vi "RP Lockin Fast Continuous Sweeper.vi"(6 "Samples per read":i32=1024, 7 "Desimate result":i32, 8 "Error In":errorcluster, 10 "Frequencies":dbl[](array[numeric]), 11 "connection ID":refnum<k5>) -> (0 "Error Out":errorcluster, 1 "Y":dbl[](array[numeric]), 2 "X":dbl[](array[numeric]), 3 "connection ID out":refnum<k5>, 4 "F":dbl[](array[numeric]))   [LabVIEW 2015]
panel:
  out "Input Fifo cnt 2":i32
  out "32bit integer":i32
  out "Output Fifo cnt":i32
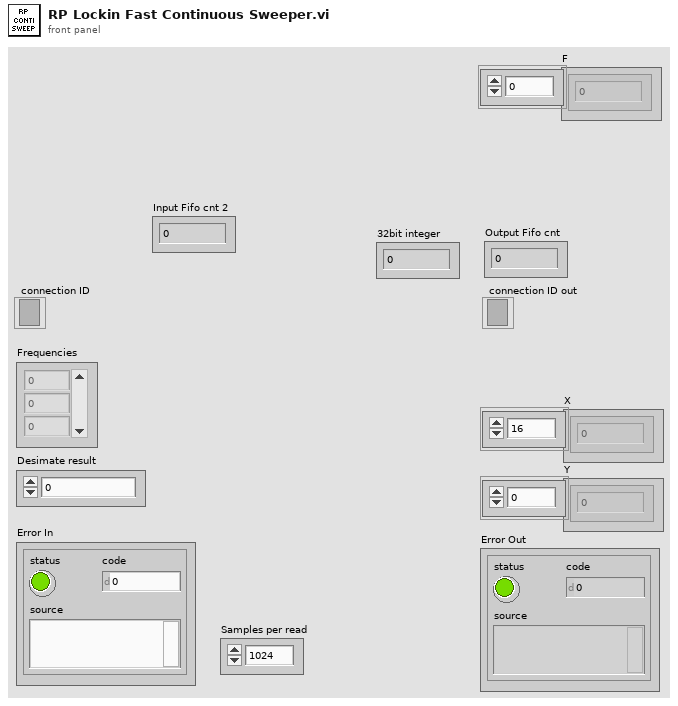
[diagram p1: front panel]
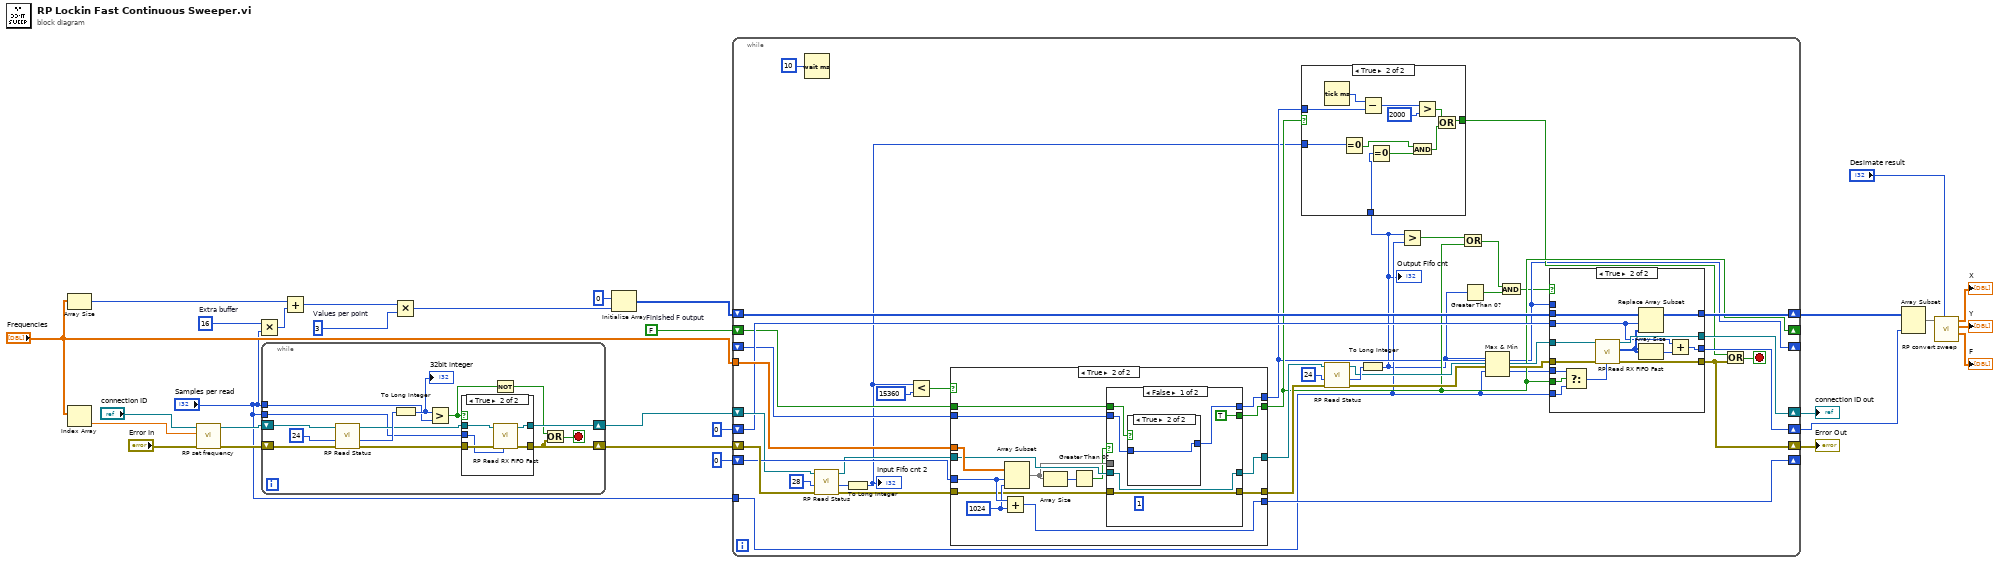
[diagram p0: block diagram]
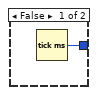
[diagram p5: hidden frame]
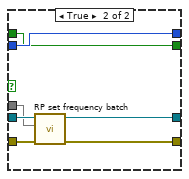
[diagram p6: hidden frame]
diagram:
  w13 = 3  # Values per point
  w16 = 16  # Extra buffer
  w19 = FALSE  # Finished F output
  n1 = Array Size(array="Frequencies") -> (size(s)=w17:i32)
  n2 = Index Array(array="Frequencies") -> (element=w29:dbl)  [unwired: 1 in]
  n3 = call "RP set frequency.vi"("Error In"="Error In", "Frequency"=w29, "connection ID"="connection ID") -> ("Error Out"=w23:errorcluster, "connection ID out"=w25:refnum<k5>)  [unwired: 6 in, 1 out]
  n4 = Multiply(x=w16, y="Samples per read") -> (x*y=w15:i32)
  n5 = while {
    tunnel: "Samples per read" -> [w40]
    shift-right: [w30] -> w22
    shift-left: w23 -> [w37]
    shift-right: [w35] -> w24
    shift-left: w25 -> [w36]
    tunnel: "Samples per read" -> [w34]
    stop <- w33 stop-if-true
    n6 = call "RP Read Status.vi"("Error In"=w37, "Status offset"=u64 24, "connection ID"=w36) -> ("Error Out"=w32:errorcluster, "Status response"=w41:u32, "connection ID out"=w39:refnum<k5>)  [unwired: 6 in]
    n7 = To Long Integer(number=w41) -> (32bit integer=w42:i32)
    "32bit integer" <- w42
    n8 = Greater?(x=w42, y=w40) -> (0:w38:bool)
    n9 = case shown="True" w38 {
      tunnel: w39 -> [w45 w50]
      tunnel: w32 -> [w44 w49]
      tunnel: [w44 w48] -> w30
      tunnel: [w45 w47] -> w35
      tunnel: w34 -> [_ w46]
      frame False {
      }
      frame True {
        n10 = call "RP Read RX FIFO Fast.vi"("Samples per read"=w46, "Error In"=w49, "connection ID"=w50) -> ("Error Out"=w48:errorcluster, "connection ID out"=w47:refnum<k5>)  [unwired: 6 in, 1 out]
      }
    }
    n11 = Not(x=w38) -> (.not. x?=w31:bool)
    n12 = Or(x=w31, y=w30) -> (x .or. y?=w33:bool)
  }
  n13 = Add(x=w17, y=w15) -> (x+y=w14:i32)
  n14 = Multiply(x=w14, y=w13) -> (x*y=w11:i32)
  n15 = Initialize Array(0, w11) -> (w10:i32[])
  n16 = while {
    tunnel: "Frequencies" -> [w88]
    tunnel: "Samples per read" -> [w53]
    shift-right: [w62] -> w20
    shift-left: w22 -> [w87]
    shift-right: [w86] -> w26
    shift-left: w24 -> [w70]
    shift-right: [w83] -> _
    shift-left: 0 -> [w84]
    shift-right: [w59] -> _
    shift-left: w19 -> [w60]
    shift-right: [w65] -> w8
    shift-left: w10 -> [w68]
    shift-right: [w66] -> w5
    shift-left: 0 -> [w67]
    shift-right: [w57] -> _
    shift-left: _ -> [w61]
    stop <- w85 stop-if-true
    n17 = Wait (ms)(milliseconds to wait=u32 10) -> ()  [unwired: 1 out]
    n18 = call "RP Read Status.vi"("Error In"=w87, "Status offset"=u64 28, "connection ID"=w70) -> ("Error Out"=w74:errorcluster, "Status response"=w78:u32, "connection ID out"=w73:refnum<k5>)  [unwired: 6 in]
    n19 = To Long Integer(number=w78) -> (32bit integer=w51:i32)
    "Input Fifo cnt 2" <- w51
    n20 = Less?(x=w51, y=15360) -> (x < y?=w75:bool)
    n21 = case shown="True" w75 {
      tunnel: w84 -> [w105 w119]
      tunnel: w88 -> [_ w120]
      tunnel: [w105 w117] -> w83
      tunnel: w74 -> [w103 w115]
      tunnel: w73 -> [w104 w114]
      tunnel: [w104 w113] -> w72
      tunnel: [w103 w112] -> w71
      tunnel: [w102 w109] -> w57
      tunnel: w61 -> [w102 w108]
      tunnel: w60 -> [w101 w107]
      tunnel: [w101 w106] -> w59
      frame False {
      }
      frame True {
        w118 = 1024
        n22 = Add(x=w119, y=w118) -> (x+y=w117:i32)
        n23 = Array Subset(array=w120, index=w119, length=w118) -> (w111:dbl[])
        n24 = Array Size(array=w111) -> (size(s)=w116:i32)
        n25 = Greater Than 0?(x=w116) -> (x > 0?=w110:bool)
        n26 = case shown="False" w110 {
          tunnel: w115 -> [w126 w135]
          tunnel: w114 -> [w125 w134]
          tunnel: [w125 w133] -> w113
          tunnel: [w126 w132] -> w112
          tunnel: w111 -> [_ w131]
          tunnel: [w124 w130] -> w109
          tunnel: w108 -> [w123 w130]
          tunnel: w107 -> [w122 w129]
          tunnel: [TRUE w129] -> w106
          frame False {
            (unwired) 1
            n27 = case shown="True" w122 {
              tunnel: [w127 w128] -> w124
              tunnel: w123 -> [_ w128]
              frame False {
                n28 = Tick Count (ms)() -> (millisecond timer value=w127:u32)
              }
              frame True {
              }
            }
          }
          frame True {
            n29 = call "RP set frequency batch.vi"("Error In"=w135, "Frequency"=w131, "connection ID"=w134) -> ("Error Out"=w132:errorcluster, "connection ID out"=w133:refnum<k5>)  [unwired: 7 in]
          }
        }
      }
    }
    n30 = call "RP Read Status.vi"("Error In"=w71, "Status offset"=u64 24, "connection ID"=w72) -> ("Error Out"=w79:errorcluster, "Status response"=w81:u32, "connection ID out"=w80:refnum<k5>)  [unwired: 6 in]
    n31 = To Long Integer(number=w81) -> (32bit integer=w52:i32)
    "Output Fifo cnt" <- w52
    n32 = case shown="True" w59 {
      selector: w59 -> [w89 _]
      tunnel: [w89 w91] -> w58
      tunnel: w57 -> [_ w96]
      tunnel: w52 -> [_ w95]
      tunnel: w51 -> [_ w94]
      frame False {
      }
      frame True {
        n33 = Tick Count (ms)() -> (millisecond timer value=w98:u32)
        n34 = Equal To 0?(x=w94) -> (x = 0?=w93:bool)
        n35 = Subtract(x=w98, y=w96) -> (x-y=w99:u32)
        n36 = Equal To 0?(x=w95) -> (x = 0?=w92:bool)
        n37 = And(x=w93, y=w92) -> (x .and. y?=w90:bool)
        n38 = Greater?(x=w99, y=u32 2000) -> (0:w97:bool)
        n39 = Or(x=w97, y=w90) -> (x .or. y?=w91:bool)
      }
    }
    n40 = Greater?(x=w52, y=w53) -> (0:w63:bool)
    n41 = Or(x=w63, y=w59) -> (x .or. y?=w64:bool)
    n42 = Greater Than 0?(x=w52) -> (x > 0?=w55:bool)
    n43 = Max & Min(x=w52, y=w53) -> (min(x,y)=w54:i32)  [unwired: 1 out]
    n44 = And(x=w64, y=w55) -> (x .and. y?=w56:bool)
    n45 = case shown="True" w56 {
      tunnel: w80 -> [w138 w153]
      tunnel: w79 -> [w139 w151]
      tunnel: [w139 w150] -> w62
      tunnel: [w138 w152] -> w86
      tunnel: w68 -> [w137 w149]
      tunnel: w67 -> [w136 w143]
      tunnel: [w136 w141] -> w66
      tunnel: [w137 w147] -> w65
      tunnel: w53 -> [_ w144]
      tunnel: w54 -> [_ w145]
      tunnel: w59 -> [_ w140]
      tunnel: w57 -> [_ _]
      frame False {
      }
      frame True {
        n46 = Select(t=w145, s=w140, f=w144) -> (s? t:f=w146:i32)
        n47 = call "RP Read RX FIFO Fast.vi"("Samples per read"=w146, "Error In"=w151, "connection ID"=w153) -> ("Error Out"=w150:errorcluster, "FIFO out"=w148:i32[], "connection ID out"=w152:refnum<k5>)  [unwired: 6 in]
        n48 = Replace Array Subset(array=w149, new element=w148, index=w143) -> (w147:i32[])
        n49 = Array Size(array=w148) -> (size(s)=w142:i32)
        n50 = Add(x=w143, y=w142) -> (x+y=w141:i32)
      }
    }
    n51 = Or(x=w58, y=w62) -> (x .or. y?=w85:bool)
  }
  "connection ID out" <- w26
  "Error Out" <- w20
  n52 = Array Subset(array=w8, length=w5) -> (w6:i32[])  [unwired: 1 in]
  n53 = call "RP convert sweep.vi"("Desimate result"="Desimate result", "FIFO"=w6) -> ("F out"=→"F":dbl[], "Y out"=→"Y":dbl[], "X out"=→"X":dbl[])  [unwired: 7 in]
